vi "Untitled 1.vi"() -> ()   [LabVIEW 2016]
panel:
  out "Waveform Graph":dbl[](graph)
  out "Boolean 3":bool
  out "Boolean 2":bool
  out "Boolean":bool
  in  "Dial":dbl(knob) scale=0.0..10.0
  in  "Numeric":dbl
  in  "stop (F)":bool
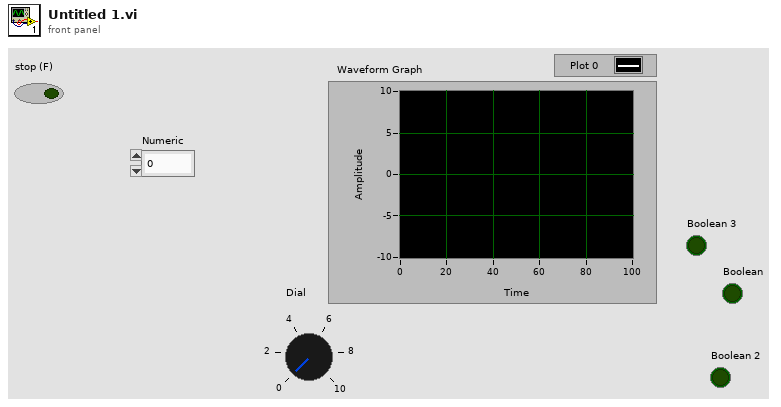
[diagram p1: front panel]
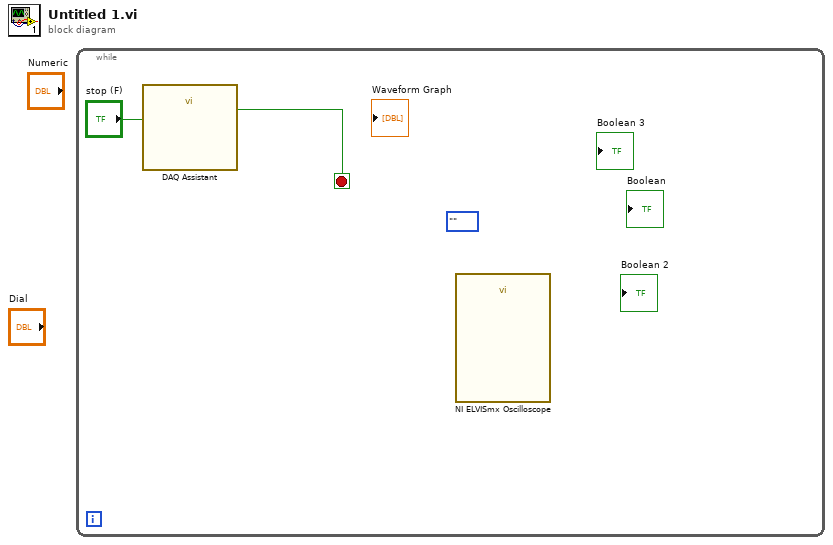
[diagram p0: block diagram]
diagram:
  n1 = while {
    stop <- w1 stop-if-true
    (unwired) enum16{""}.""
    n2 = call "DAQ Assistant"("stop (F)"="stop (F)") -> ("stopped"=w1:bool)  [unwired: 15 in, 3 out]
    n3 = call "NI ELVISmx Oscilloscope"() -> ()  [unwired: 17 in, 3 out]
  }
